vi "Dual XDCR Scan.vi"(0 "Digitizer Settings In":T27={"Digitizer delay (us) "=0.0, "rf points per line"=0, "lines per plane"=0, "Samp Rate (Hz)"=0.0, "Additional dig delay (us)"=0.0, "Voltage Scale"=0.0, "Pre-Looks"=0, "Offset delay (us)"=0.0, "bits A/D"=0, "Avg Num"=0, "DigTimeOut"=0.0, "Rel Dig Delay"=0.0, "Dig Ch"=0, "LeCroyCluster"={"LeCroy Channels"=[], "LC read pt offset"=0.0, "Sweep Avg"=FALSE}, "Main Digitizer"=enum."Acqiris Digitizer", "Dig Config"=enum."Single channel", "Digitizer ID Cluster"={"Acqiris/Alazar/SP ID"=[], "NI Instr Handles"=[], "LeCroy VISA"="", "GaGe Handle"={"Handle"=0, "Sample size"=0, "Resolution"=0, "Offset"=0, "Channels"=0, "Boards"=0}, "ATS Ref"="ATS9350", "Acqiris Address"=["PCI::INSTR0"], "ADQRef"=refnum, "adq_cu_ptr"=refnum}, "Trigger Settings"={"Trig Source"=0, "Trig Coupling"=0, "Trig Slope"=0, "Level (mV)"=0.0}, "Bulk Acq"=FALSE, "Bulk Start Indexes"=[], "Data Ref RF"=refnum, "NI ID/Channel"=[], "Total Dig CH"=1, "Xtra Ann Trig delay (us)"=10.0, "Fix Z Delay?"=FALSE, "One Way Transmission?"=FALSE, "Data Ref Log"=refnum} {"Trigger Settings"."Trig Slope" items=["Positive", "Negative"]; "Trigger Settings"."Level (mV)" format="%.2f"; "Trigger Settings"."Trig Coupling" items=["DC 1 MOhm", "AC 1 MOhm", "DC 50 Ohm", "AC 50 Ohm"]; "Trigger Settings"."Trig Source" items=["Chan 1", "External"]; "Rel Dig Delay" format="%.2f"; "DigTimeOut" format="%.2f"; "Avg Num" min=1; "Offset delay (us)" format="%.2f"; "Additional dig delay (us)" format="%.2f"; "Digitizer delay (us)" format="%.2f"}, 1 "Dual XDCR Mode":T36(ring)=enum."Exit", 3 "Motion Settings In":T31={"No Motion?"=FALSE, "Motion System"=enum."MM3000", "Motion Bd ID"=0, "Motion Profile"="SMAC1", "# Axis"=0, "Reverse Z axis?"=FALSE, "SMAC Axis"=0, "scan pair"=enum."y-(x) scan", "RT fps"=0.0, "Steps per mm"=[], "Motor Parameters"={"velocity ct/s"=[], "accel ct/s^2"=[]}, "One Way Scan"=FALSE, "Reverse One Way Scan"=FALSE, "Global Position (mm)"=[], "Plane"=0, "Distance between\nscan lines (um)"=0.0, "Distance between\nscan planes (um)"=0.0, "number of scan planes"=0, "Total steps in line"=0, "Xtra plane\ndistance  (um)"=0, "Xtra planes "=0, "Add Axis"=FALSE, "overshoot cts"=0, "BKPT Shift"=0, "Scan Start Time (ms)"=0, "ESP VISA"="", "3rd Axis"=1, "GL Ref Out"=refnum, "Galil Address"=""} {"3rd Axis" items=["x", "y", "z", "w"]; "Xtra planes" min=1; "Xtra plane\ndistance  (um)" min=0; "Distance between\nscan planes (um)" format="%.2f"; "Distance between\nscan lines (um)" format="%.2f"; "SMAC Axis" items=["None"=0, "Axis 1"=1, "Axis 2"=2, "Axis 3"=3, "Axis 4"=4, "Axis 5"=5, "Axis 6"=6, "Axis 7"=7, "Axis 8"=8, "Vector Space 1"=17, "Vector Space 2"=18, "Vector Space 3"=19, "Vector Space 4"=20]; "Motion Bd ID" min=1 max=32 step=1}, 5 "Switch Unit":T35=enum."Riverside USB", 6 "Ann Array Params":T23={"Synth Foc?"=FALSE, "Focal Zones"=41, "Switch T/R"=0, "Trans Geometry (mm)"={"Transducer"=0, "Geo Focus"=12.0, "a (radius)"=3.0, "# of rings"=5, "kerf space "=0.1, "Center Freq"=12.0}, "Sub Ap Excite?"=FALSE, "Full Array Scan?"=FALSE, "Xmt/Rcv"={"XMIT"=[TRUE, TRUE, TRUE, TRUE, TRUE], "RCV"=[TRUE, TRUE, TRUE, TRUE, TRUE]}, "PulseSpacing (us)"=0.0, "Xmit Ring"=0, "XMIT CHS"=0, "RCV CHS"=0, "GPU?"=FALSE, "Save TIFF?"=FALSE, "downfactor"=1, "RCV 1CH"=0} {"RCV 1CH" items=["All", "1", "2", "3", "4", "5"]; "Trans Geometry (mm)"."Transducer" items=["6D 12R 40 MHz"=0, "10D 31R 20 MHz"=1, "10D 23R 20 MHz"=2, "6D 23R 40 MHz"=3, "4.5D 10.7R 40 MHz"=4, "9D 23.5R 20 MHz"=5, "9D 25.8R 20MHz"=6, "Enter"=99]; "Switch T/R" min=1 max=5 step=1}, 7 "Case Name":string, 8 "Scan Parameters  Cluster":T1, 9 "Dual XDCR Settings":T2 {"XDCR Settings"."UT340 Controls"."Low Pass Filter (MHz)" min=-6 max=60 step=1; "XDCR Settings"."UT340 Controls"."High Pass Filter (MHz)" min=1 max=20 step=1; "XDCR Settings"."UT340 Controls"."Rep Rate (Hz)" min=20 step=1; "XDCR Settings"."UT340 Controls"."Pulse Width (ns)" min=100.0 max=250.0 step=2.0; "XDCR Settings"."UT340 Controls"."Voltage" min=100 max=250 step=2; "XDCR Settings"."UT340 Controls"."PC Gain (dB)" min=2 max=72; "XDCR Settings"."UT340 Controls"."PE Gain (dB)" min=-6 max=60 step=1; "XDCR Settings"."JSR Complete"."JSR Trigger Settings"."PRF (Hz)" items=["100 Hz"=0.1, "200 Hz"=0.2, "400 Hz"=0.4, "600 Hz"=0.6, "800 Hz"=0.8, "1000 Hz"=1.0, "1250 Hz"=1.25, "1500 Hz"=1.5, "1750 Hz"=1.75, "2000 Hz"=2.0, "2500 Hz"=2.5, "3000 Hz"=3.0, "3500 Hz"=3.5, "4000 Hz"=4.0, "4500 Hz"=4.5, "5000 Hz"=5.0]; "XDCR Settings"."JSR Complete"."JSR Trigger Settings"."Trigger Source" items=["Internal", "External"]; "XDCR Settings"."JSR Complete"."JSR Trigger Settings"."External Trigger Limit" items=["No Limit", "5 kHz"]; "XDCR Settings"."JSR Complete"."JSR Receive Settings"."Gain (dB)" min=-13 max=66 step=1; "XDCR Settings"."JSR Complete"."JSR Receive Settings"."Low Pass Filter" items=["5 MHz"=5, "10 MHz"=10, "15 MHz"=15, "22.5 MHz"=22, "35 MHz"=35, "50 MHz"=50]; "XDCR Settings"."JSR Complete"."JSR Receive Settings"."High Pass Filter" items=["DC"=0, "1 MHz"=1000, "2.5 MHz"=2500, "5 MHz"=5000, "7.5 MHz"=7500, "12.5 MHz"=12500]; "XDCR Settings"."JSR Complete"."JSR Receive Settings"."Receiver Mode" items=["Echo", "Through"]; "XDCR Settings"."JSR Complete"."JSR Pulse Settings"."Pulser Voltage (V)" items=["100"=100, "125"=125, "150"=150, "175"=175, "200"=200, "225"=225, "250"=250, "275"=275, "300"=300, "325"=325, "350"=350, "375"=375, "400"=400, "425"=425, "450"=450, "475"=475]; "XDCR Settings"."JSR Complete"."JSR Pulse Settings"."Pulser Impedance" items=["High z", "Low z"]; "XDCR Settings"."JSR Complete"."JSR Pulse Settings"."Pulse Energy Level" items=["0 (Minimum)", "1", "2", "3 (Maximum)"]; "XDCR Settings"."JSR Complete"."JSR Pulse Settings"."Damping" items=["331 Ohms"=331, "198 Ohms"=198, "142 Ohms"=142, "110 Ohms"=110, "92 Ohms"=92, "77 Ohms"=77, "67 Ohms"=67, "59 Ohms"=59, "52 Ohms"=52, "47 Ohms"=47, "43 Ohms"=43, "39 Ohms"=39, "37 Ohms"=37, "34 Ohms"=34, "32 Ohms"=32, "30 Ohms"=30]; "XDCR Settings"."Panametrics Settings"."FINE ATTENUATION" items=["00.0", "00.5", "01.0", "01.5", "02.0", "02.5", "03.0", "03.5", "04.0", "04.5", "05.0", "05.5", "06.0", "06.5", "07.0", "07.5", "08.0", "08.5", "09.0", "09.5", "10.0", "10.5", "11.0", "11.5", "12.0", "12.5", "13.0", "13.5", "14.0", "14.5", "15.0", "15.5"]; "XDCR Settings"."Panametrics Settings"."COARSE ATTENUATION" items=["00.0", "10.0", "20.0", "30.0", "40.0", "50.0"]; "XDCR Settings"."Panametrics Settings"."GAIN (db)" items=["26.0", "40.0", "54.0"]; "XDCR Settings"."Panametrics Settings"."PRF (KHz)" items=["XREMT", "EXBNC", "0.200", "0.500", "1.000", "2.000", "5.000", "10.00", "20.00"]; "XDCR Settings"."Panametrics Settings"."MODE" items=["P/ E", "THRU", "RPP", "EXT_PLSR"]; "XDCR Settings"."Panametrics Settings"."LP FILT (MHz)" items=["20", "50", "100", "200"]; "XDCR Settings"."Panametrics Settings"."HP FILT (KHz)" items=["1", "1000", "3000", "10000"]; "XDCR Settings"."Panametrics Settings"."DAMPING (Ohm)" items=["7", "10", "16", "20", "26", "30", "40", "50"]; "XDCR Settings"."Panametrics Settings"."ENERGY (uJ)" items=["1", "2", "4", "8", "16", "32"]; "XDCR Settings"."Daxsonics Settings"."Freq (MHz)" items=["4"=4, "5"=5, "6"=6, "8"=8, "10"=10, "12"=12, "14"=14, "15"=15, "16"=16, "17"=17, "18"=18, "20"=20, "25"=25, "30"=30, "35"=35, "40"=40, "45"=45, "50"=50]; "XDCR Settings"."Daxsonics Settings"."Voltage (V)" items=["0"=0, "5"=5, "10"=10, "15"=15, "20"=20, "25"=25, "30"=30, "35"=35, "40"=40, "45"=45, "50"=50, "55"=55, "60"=60, "65"=65, "70"=70, "75"=75, "80"=80, "85"=85, "90"=90, "95"=95, "100"=100, "110"=110, "120"=120, "130"=130, "140"=140, "150"=150, "160"=160, "170"=170, "180"=180, "190"=190]; "XDCR Settings"."Daxsonics Settings"."Gain (dB)" items=["22"=22, "25"=25, "28"=28, "31"=31, "34"=34, "37"=37, "40"=40, "43"=43, "46"=46, "49"=49, "52"=52, "55"=55, "58"=58, "61"=61, "64"=64, "67"=67]; "XDCR Settings"."Digitizer Settings"."Additional dig delay (ms)" format="%.2f"; "XDCR Settings"."Digitizer Settings"."Time scale per Div" items=["100 ns"=0.1, "200 ns"=0.2, "500 ns"=0.5, "1 micros"=1.0, "2 micros"=2.0, "5 micros"=5.0, "10 micros"=10.0, "20 micros"=20.0, "50 micros"=50.0, "100 micros"=100.0, "200 micros"=200.0, "500 micros"=500.0, "1 ms"=1000.0, "2 ms"=2000.0, "5 ms"=5000.0, "10 ms"=10000.0, "20 ms"=20000.0, "50 ms"=50000.0, "100 ms"=100000.0, "200 ms"=200000.0]; "XDCR Settings"."Digitizer Settings"."RF data Sampling"."rf points per line" min=1; "XDCR Settings"."Digitizer Settings"."RF data Sampling"."Ref Delay (ms)" format="%.2f"}) -> (12 "Ann Array Params":T23={"Synth Foc?"=FALSE, "Focal Zones"=41, "Switch T/R"=0, "Trans Geometry (mm)"={"Transducer"=0, "Geo Focus"=12.0, "a (radius)"=3.0, "# of rings"=5, "kerf space "=0.1, "Center Freq"=12.0}, "Sub Ap Excite?"=FALSE, "Full Array Scan?"=FALSE, "Xmt/Rcv"={"XMIT"=[TRUE, TRUE, TRUE, TRUE, TRUE], "RCV"=[TRUE, TRUE, TRUE, TRUE, TRUE]}, "PulseSpacing (us)"=0.0, "Xmit Ring"=0, "XMIT CHS"=0, "RCV CHS"=0, "GPU?"=FALSE, "Save TIFF?"=FALSE, "downfactor"=1, "RCV 1CH"=0} {"RCV 1CH" items=["All", "1", "2", "3", "4", "5"]; "Trans Geometry (mm)"."Transducer" items=["6D 12R 40 MHz"=0, "10D 31R 20 MHz"=1, "10D 23R 20 MHz"=2, "6D 23R 40 MHz"=3, "4.5D 10.7R 40 MHz"=4, "9D 23.5R 20 MHz"=5, "9D 25.8R 20MHz"=6, "Enter"=99]; "Switch T/R" min=1 max=5 step=1}, 13 "Case Names":string[](array[string]), 14 "Digitizer Settings":T27={"Digitizer delay (us) "=0.0, "rf points per line"=2048, "lines per plane"=128, "Samp Rate (Hz)"=100000000.0, "Additional dig delay (us)"=0.0, "Voltage Scale"=0.4, "Pre-Looks"=0, "Offset delay (us)"=0.0, "bits A/D"=8, "Avg Num"=1, "DigTimeOut"=5.0, "Rel Dig Delay"=0.0, "Dig Ch"=0, "LeCroyCluster"={"LeCroy Channels"=[TRUE, FALSE, FALSE, FALSE], "LC read pt offset"=0.0, "Sweep Avg"=FALSE}, "Main Digitizer"=enum."NI Digitizer", "Dig Config"=enum."Single channel", "Digitizer ID Cluster"={"Acqiris/Alazar/SP ID"=[], "NI Instr Handles"=[], "LeCroy VISA"="", "GaGe Handle"={"Handle"=0, "Sample size"=0, "Resolution"=0, "Offset"=0, "Channels"=0, "Boards"=0}, "ATS Ref"="ATS9350", "Acqiris Address"=["PCI::INSTR0"], "ADQRef"=refnum, "adq_cu_ptr"=refnum}, "Trigger Settings"={"Trig Source"=1, "Trig Coupling"=0, "Trig Slope"=0, "Level (mV)"=1500.0}, "Bulk Acq"=FALSE, "Bulk Start Indexes"=[], "Data Ref RF"=refnum, "NI ID/Channel"=[], "Total Dig CH"=1, "Xtra Ann Trig delay (us)"=10.0, "Fix Z Delay?"=FALSE, "One Way Transmission?"=FALSE, "Data Ref Log"=refnum} {"Trigger Settings"."Trig Slope" items=["Positive", "Negative"]; "Trigger Settings"."Level (mV)" format="%.2f"; "Trigger Settings"."Trig Coupling" items=["DC 1 MOhm", "AC 1 MOhm", "DC 50 Ohm", "AC 50 Ohm"]; "Trigger Settings"."Trig Source" items=["Chan 1", "External"]; "Rel Dig Delay" format="%.2f"; "DigTimeOut" format="%.2f"; "Avg Num" min=1; "Offset delay (us)" format="%.2f"; "Additional dig delay (us)" format="%.2f"; "Digitizer delay (us)" format="%.2f"}, 15 "Error Message":string, 17 "Motion Settings":T31={"No Motion?"=FALSE, "Motion System"=enum."NI 735x", "Motion Bd ID"=1, "Motion Profile"="SMAC1", "# Axis"=1, "Reverse Z axis?"=TRUE, "SMAC Axis"=0, "scan pair"=enum."y-(x) scan", "RT fps"=6.0, "Steps per mm"=[1000, 1000, 1000, 1000], "Motor Parameters"={"velocity ct/s"=[10000.0, 10000.0, 10000.0, 50000.0], "accel ct/s^2"=[50000.0, 50000.0, 50000.0, 200000.0]}, "One Way Scan"=FALSE, "Reverse One Way Scan"=FALSE, "Global Position (mm)"=[], "Plane"=0, "Distance between\nscan lines (um)"=0.0, "Distance between\nscan planes (um)"=0.0, "number of scan planes"=1, "Total steps in line"=0, "Xtra plane\ndistance  (um)"=100, "Xtra planes "=1, "Add Axis"=FALSE, "overshoot cts"=200, "BKPT Shift"=0, "Scan Start Time (ms)"=0, "ESP VISA"="GPIB::1::INSTR", "3rd Axis"=1, "GL Ref Out"=refnum, "Galil Address"=""} {"3rd Axis" items=["x", "y", "z", "w"]; "Xtra planes" min=1; "Xtra plane\ndistance  (um)" min=0; "Distance between\nscan planes (um)" format="%.2f"; "Distance between\nscan lines (um)" format="%.2f"; "SMAC Axis" items=["None"=0, "Axis 1"=1, "Axis 2"=2, "Axis 3"=3, "Axis 4"=4, "Axis 5"=5, "Axis 6"=6, "Axis 7"=7, "Axis 8"=8, "Vector Space 1"=17, "Vector Space 2"=18, "Vector Space 3"=19, "Vector Space 4"=20]; "Motion Bd ID" min=1 max=32 step=1}, 18 "Scan Params Array":T26[](array[typedef]), 19 "Num Scans":i32)   [LabVIEW 2022 SP3]
uses:
  Motion Controllers/NI_controller/-NI_MotionRoutines/MotionParameters.ctl
  Motion Controllers/NI_controller/-NI_MotionRoutines/MotionSys.ctl
  Motion Controllers/-MotionRoutines/ScanAxis.ctl
  Motion Controllers/-MotionRoutines/3rdAxis.ctl
  Digitizers/-DigitizerRoutines/DigitizerSettings.ctl
  Digitizers/-DigitizerRoutines/Digitizer.ctl
  Digitizers/-DigitizerRoutines/DigConfig.ctl
  Digitizers/-DigitizerRoutines/DigitizerID.ctl
  C:/Windows/System32/ADQAPI_dotNet_helper.dll
  Switch Modules/SwitchOption.ctl
  -ScanSystem/Controls/ScanParams.ctl
  Annular Array/-AnnularRoutines/AnnularArray.ctl
  Annular Array/-AnnularRoutines/TransGeometry.ctl
  Annular Array/-AnnularRoutines/ArrayGeometry.ctl
  -ScanSystem/Controls/location.ctl
  Dual XDCR Complete Settings.ctl
  XDCRSettings.ctl
  Pulsers/Daxsonics/-DaxSubroutines/Dax_Control_Cluster.ctl
  Pulsers/Panametrics/Pana5900.ctl
  Pulsers/JSR/Controls/JSR Complete.ctl
  Pulsers/JSR/Controls/JSR Pulse.ctl
  Pulsers/JSR/Controls/Damping.ctl
  Pulsers/JSR/Controls/Energy.ctl
  Pulsers/JSR/Controls/Z.ctl
  Pulsers/JSR/Controls/Volt.ctl
  Pulsers/JSR/Controls/JSR Recieve.ctl
  Pulsers/JSR/Controls/Mode.ctl
  Pulsers/JSR/Controls/HPF.ctl
  Pulsers/JSR/Controls/LPF.ctl
  Pulsers/JSR/Controls/Gain.ctl
  Pulsers/JSR/Controls/JSR Trigger.ctl
  Pulsers/JSR/Controls/Trig Limit.ctl
  Pulsers/JSR/Controls/Trig Source.ctl
  Pulsers/JSR/Controls/PRF.ctl
  Pulsers/UTEX/Controls/UTEX Controls.ctl
  -ScanSystem/Controls/ScanType2.ctl
  Motion Controllers/-MotionRoutines/MotionGlobals.vi
  Pulsers/PulserGlobals.vi
  <instrlib>/niSwitch/niSwitch.llb/niSwitch Connect Channels (Single).vi
panel:
  out "Location":T22=enum."WCM Main"
  out "One Way Scan":bool
  # "1-D and 2-D B scan settings"
  # "1-D and 2-D B scan settings"
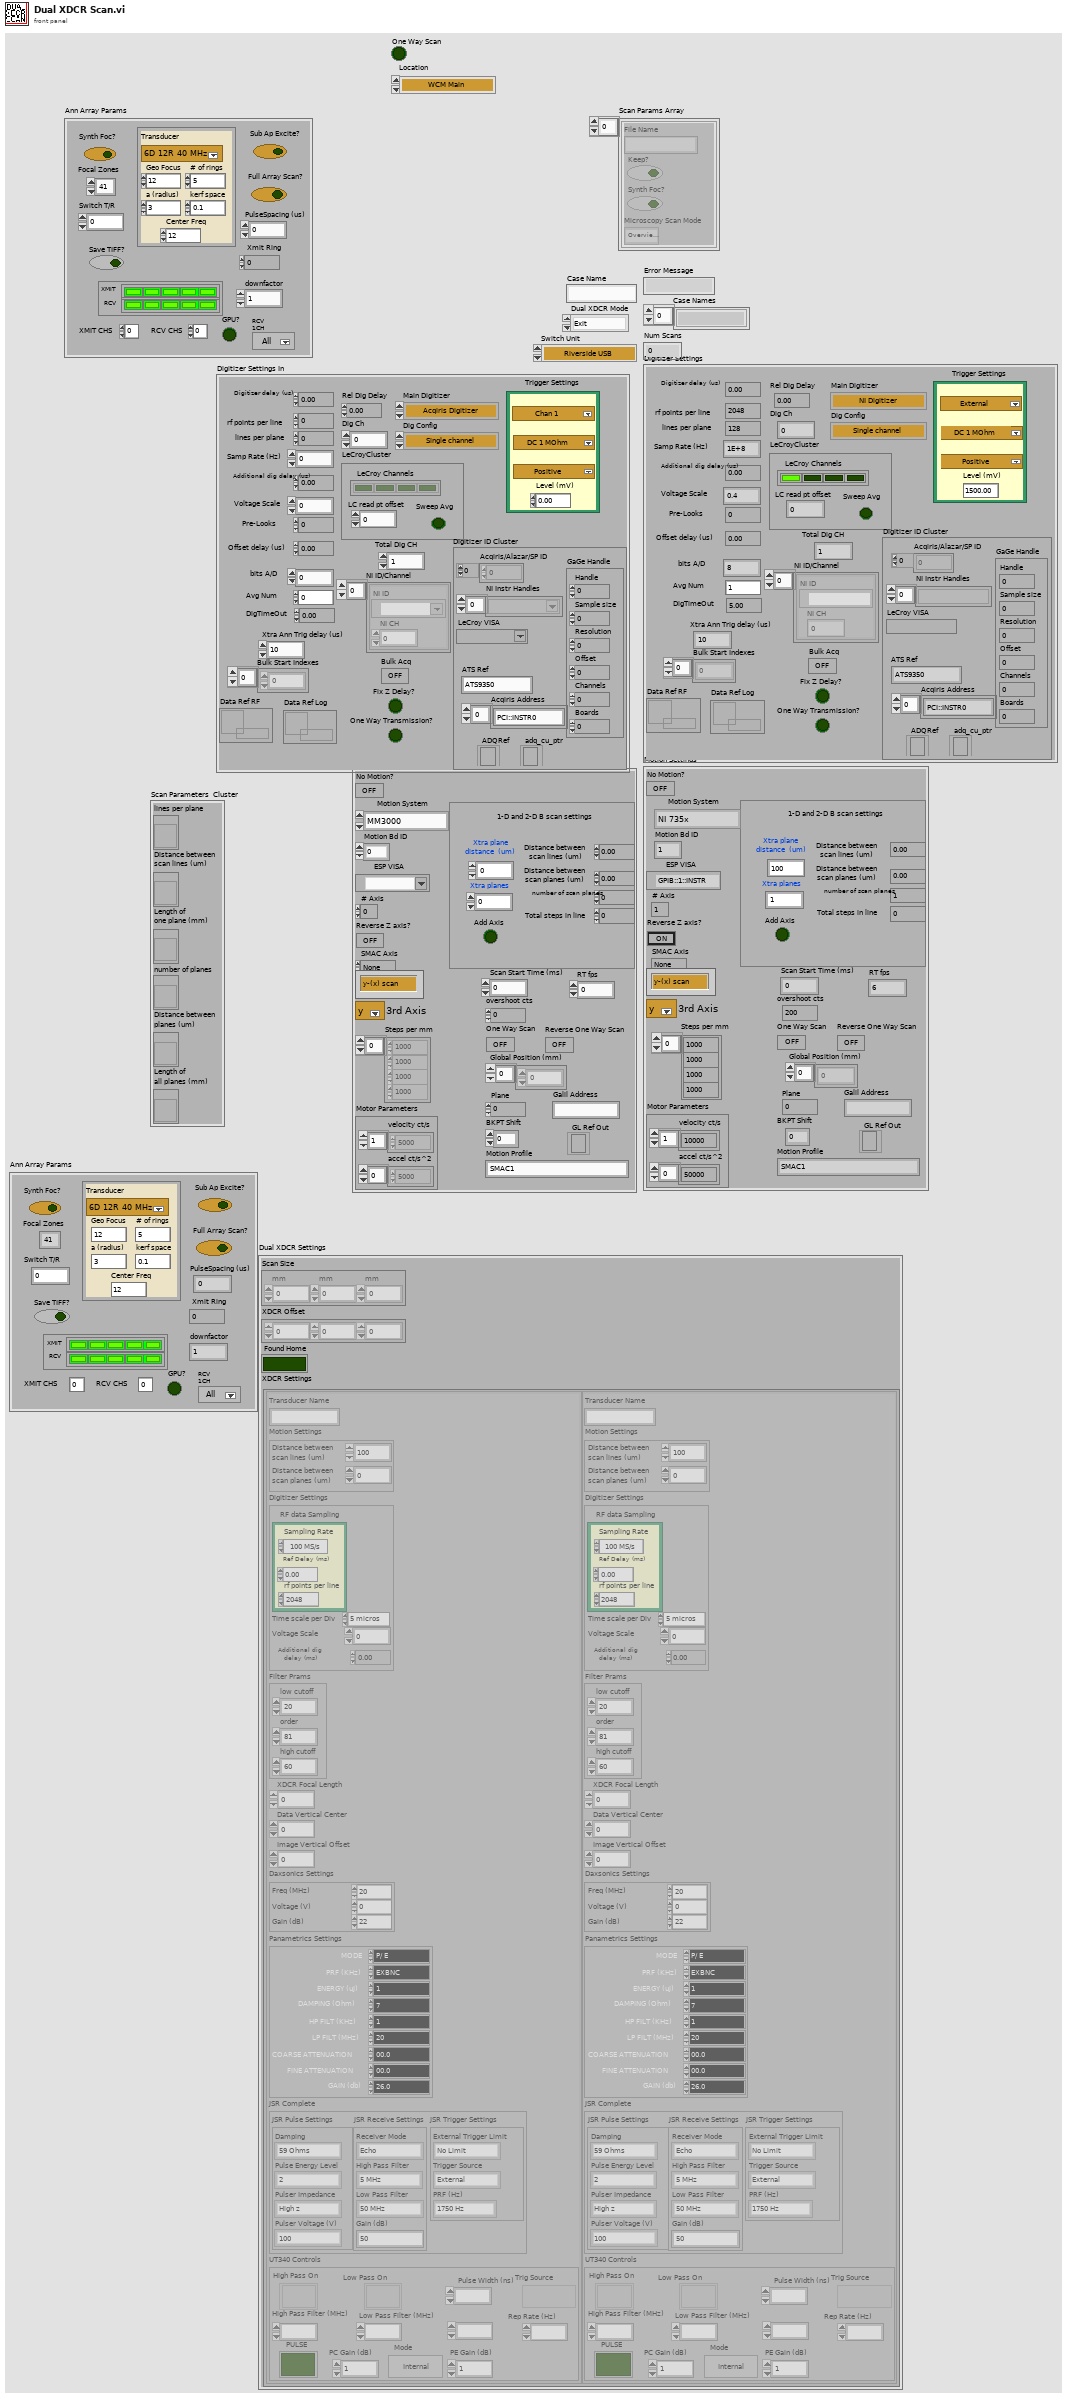
[diagram p1: front panel]
types:
  T1 = cluster{"lines per plane":refnum<vi>, "Distance between\nscan lines (um)":refnum<vi>, "Length of\none plane (mm)":refnum<vi>, "number of planes":refnum<vi>, "Distance between\nplanes (um)":refnum<vi>, "Length of\nall planes (mm)":refnum<vi>}
  T2 = typedef "Dual XDCR Complete Settings.ctl" = cluster{"Scan Size":dbl[], "XDCR Offset":dbl[], "Found Home":bool, "XDCR Settings":T3[]}
  T3 = typedef "XDCRSettings.ctl" = cluster{"Transducer Name":string, "Motion Settings":cluster{"Distance between\nscan lines (um)":sgl, "Distance between\nscan planes (um)":sgl}, "Digitizer Settings":cluster{"RF data Sampling":cluster{"Sampling Rate":dbl, "Ref Delay (ms)":dbl, "rf points per line":i32}, "Time scale per Div":dbl, "Voltage Scale":dbl, "Additional dig delay (ms)":dbl}, "Filter Prams":cluster{"low cutoff":i32, "order":i32, "high cutoff":i32}, "XDCR Focal Length":dbl, "Data Vertical Center":dbl, "Image Vertical Offset":dbl, "Daxsonics Settings":T4, "Panametrics Settings":T5, "JSR Complete":T6, "UT340 Controls":T21}
  T4 = typedef "Dax_Control_Cluster.ctl" = cluster{"Freq (MHz) ":u16, "Voltage (V)":u16, "Gain (dB)":u16}
  T5 = typedef "Pana5900.ctl" = cluster{"ENERGY (uJ)":u16, "DAMPING (Ohm)":u16, "HP FILT (KHz) ":u16, "LP FILT (MHz)":u16, "MODE":u16, "PRF (KHz)":u16, "GAIN (db)":u16, "COARSE ATTENUATION":u16, "FINE ATTENUATION":u16}
  T6 = typedef "JSR Complete.ctl" = cluster{"JSR Pulse Settings":T7, "JSR Receive Settings":T12, "JSR Trigger Settings":T17}
  T7 = typedef "JSR Pulse.ctl" = cluster{"Damping":T8, "Pulse Energy Level":T9, "Pulser Impedance":T10, "Pulser Voltage (V)":T11}
  T8 = typedef "Damping.ctl" = i16
  T9 = typedef "Energy.ctl" = u16
  T10 = typedef "Z.ctl" = u16
  T11 = typedef "Volt.ctl" = i16
  T12 = typedef "JSR Recieve.ctl" = cluster{"Receiver Mode":T13, "High Pass Filter":T14, "Low Pass Filter":T15, "Gain (dB)":T16}
  T13 = typedef "Mode.ctl" = i8
  T14 = typedef "HPF.ctl" = u16
  T15 = typedef "LPF.ctl" = u16
  T16 = typedef "Gain.ctl" = i8
  T17 = typedef "JSR Trigger.ctl" = cluster{"External Trigger Limit":T18, "Trigger Source":T19, "PRF (Hz)":T20}
  T18 = typedef "Trig Limit.ctl" = i8
  T19 = typedef "Trig Source.ctl" = i8
  T20 = typedef "PRF.ctl" = dbl
  T21 = typedef "UTEX Controls.ctl" = cluster{"High Pass On":bool, "High Pass Filter (MHz)":i16, "Low Pass On":bool, "Low Pass Filter (MHz)":i16, "PE Gain (dB)":i16, "Voltage":i16, "Pulse Width (ns)":dbl, "Mode":bool, "PC Gain (dB)":i16, "Trig Source":bool, "Rep Rate (Hz)":i16, "PULSE":bool}
  T22 = typedef "location.ctl" = enum16{"Automatic", "WCM Main", "Hawaii", "Columbia MM3000", "Columbia  NI System", "NYU", "RRI 2", "UHI Allen", "CUMC RT", "Chiba", "Stony Brook", "WCM Microscopy", "WCM Aeoretch", "WCM Optics Lab", "WCM Main 2Axis", "WCM Rotation", "WCM SAM SMAC", "SERI GP"}
  T23 = typedef "AnnularArray.ctl" = cluster{"Synth Foc?":bool, "Focal Zones":i16, "Switch T/R":i16, "Trans Geometry (mm)":T24, "Sub Ap Excite?":bool, "Full Array Scan?":bool, "Xmt/Rcv":cluster{"XMIT":bool[], "RCV":bool[]}, "PulseSpacing (us)":sgl, "Xmit Ring":i32, "XMIT CHS":u8, "RCV CHS":u8, "GPU?":bool, "Save TIFF?":bool, "downfactor":i32, "RCV 1CH":u16}
  T24 = typedef "TransGeometry.ctl" = cluster{"Transducer":T25, "Geo Focus":dbl, "a (radius)":dbl, "# of rings":i32, "kerf space ":dbl, "Center Freq":dbl}
  T25 = typedef "ArrayGeometry.ctl" = u16
  T26 = typedef "ScanParams.ctl" = cluster{"File Name":string, "Keep?":bool, "Synth Foc?":bool, "Microscopy Scan Mode":enum32{"Level X", "Level Y", "Overview Scan", "Detailed Scan", "V-Z Scan"}}
  T27 = typedef "DigitizerSettings.ctl" = cluster{"Digitizer delay (us) ":dbl, "rf points per line":i32, "lines per plane":i32, "Samp Rate (Hz)":dbl, "Additional dig delay (us)":dbl, "Voltage Scale":dbl, "Pre-Looks":i32, "Offset delay (us)":dbl, "bits A/D":i8, "Avg Num":i32, "DigTimeOut":sgl, "Rel Dig Delay":sgl, "Dig Ch":i32, "LeCroyCluster":cluster{"LeCroy Channels":bool[], "LC read pt offset":dbl, "Sweep Avg":bool}, "Main Digitizer":T28, "Dig Config":T29, "Digitizer ID Cluster":T30, "Trigger Settings":cluster{"Trig Source":u16, "Trig Coupling":u16, "Trig Slope":u16, "Level (mV)":dbl}, "Bulk Acq":bool, "Bulk Start Indexes":i32[], "Data Ref RF":refnum<data-value>, "NI ID/Channel":cluster{"NI ID":refnum<k15>, "NI CH":i32}[], "Total Dig CH":i32, "Xtra Ann Trig delay (us)":dbl, "Fix Z Delay?":bool, "One Way Transmission?":bool, "Data Ref Log":refnum<data-value>}
  T28 = typedef "Digitizer.ctl" = enum16{"Acqiris Digitizer", "NI Digitizer", "LeCroy", "GaGe", "AlazarTech", "No Digitizer", "Teledyne"}
  T29 = typedef "DigConfig.ctl" = enum16{"Single channel", "2 Chans w/ 2 Acqiris", "2 Chans w/ 1 Acqiris", "5-CH Pulser New", "5-CH pulser w/ ann array", "5-pass style ann array", "Empty"}
  T30 = typedef "DigitizerID.ctl" = cluster{"Acqiris/Alazar/SP ID":u32[], "NI Instr Handles":refnum<k15>[], "LeCroy VISA":refnum<visa-resource-name>, "GaGe Handle":cluster{"Handle":u32, "Sample size":u32, "Resolution":i32, "Offset":i32, "Channels":u32, "Boards":u32}, "ATS Ref":string, "Acqiris Address":string[], "ADQRef":refnum<k24>, "adq_cu_ptr":refnum<k24>}
  T31 = typedef "MotionParameters.ctl" = cluster{"No Motion?":bool, "Motion System":T32, "Motion Bd ID":u8, "Motion Profile":string, "# Axis":i8, "Reverse Z axis?":bool, "SMAC Axis":u16, "scan pair":T33, "RT fps":sgl, "Steps per mm":i32[], "Motor Parameters":cluster{"velocity ct/s":dbl[], "accel ct/s^2":dbl[]}, "One Way Scan":bool, "Reverse One Way Scan":bool, "Global Position (mm)":dbl[], "Plane":i32, "Distance between\nscan lines (um)":sgl, "Distance between\nscan planes (um)":sgl, "number of scan planes":i32, "Total steps in line":i32, "Xtra plane\ndistance  (um)":i32, "Xtra planes ":i32, "Add Axis":bool, "overshoot cts":i32, "BKPT Shift":i32, "Scan Start Time (ms)":u32, "ESP VISA":refnum<visa-resource-name>, "3rd Axis":T34, "GL Ref Out":refnum<k7>, "Galil Address":string}
  T32 = typedef "MotionSys.ctl" = enum16{"MM3000", "NI 735x", "Newport ESP", "No Motion Card", "Galil"}
  T33 = typedef "ScanAxis.ctl" = enum16{"y-(x) scan", "x-(y) scan", "z-(x) scan", "z-(y) scan", "y-(z) scan", "x-(z) scan", "w-(x) scan", "w-(y) scan", "w-(z) scan", "x-(w) scan", "y-(w) scan", "z-(w) scan"}
  T34 = typedef "3rdAxis.ctl" = u16
  T35 = typedef "SwitchOption.ctl" = enum16{"Cytex", "Pickering", "NI Switch", "No Switch", "Riverside USB"}
  T36 = enum16{"Transducer 1", "Transducer 2", "Dual XDCR", "Exit"}
  T37 = typedef "pulser.ctl" = enum16{"Pan 5900", "Daxsonics", "Agilent 33xxx", "UTEX", "JSR", "WMC Mono-Cycle", "No Pulser", "NYU AVTECH", "Tabor W1281A", "Pan 5800", "Unlisted", "Tabor WX2182B"}
  T38 = enum16{"Absolute Position", "Relative Position", "Velocity", "Relative to Cap Pos", "Modulus Position", "Absolute Contouring", "Relative Contouring"}
  T39 = typedef "ScanType2.ctl" = enum16{"Therapy With Scan", "M scan", "M Scan With Therapy Burst", "1-D B Scan", "1-D B Scan With Therapy Burst", "2-D B Scan", "2-D B Scan With Therapy Burst", "Rotational Scan", "1-D B-Scan PRF", "2-D B-Scan PRF", "Real-Time Scan", "Contrast Agents", "1-D w/ Real-Time Set Up", "Dual Transducer", "Acoustic Microscopy", "Hydrophone Scanning"}
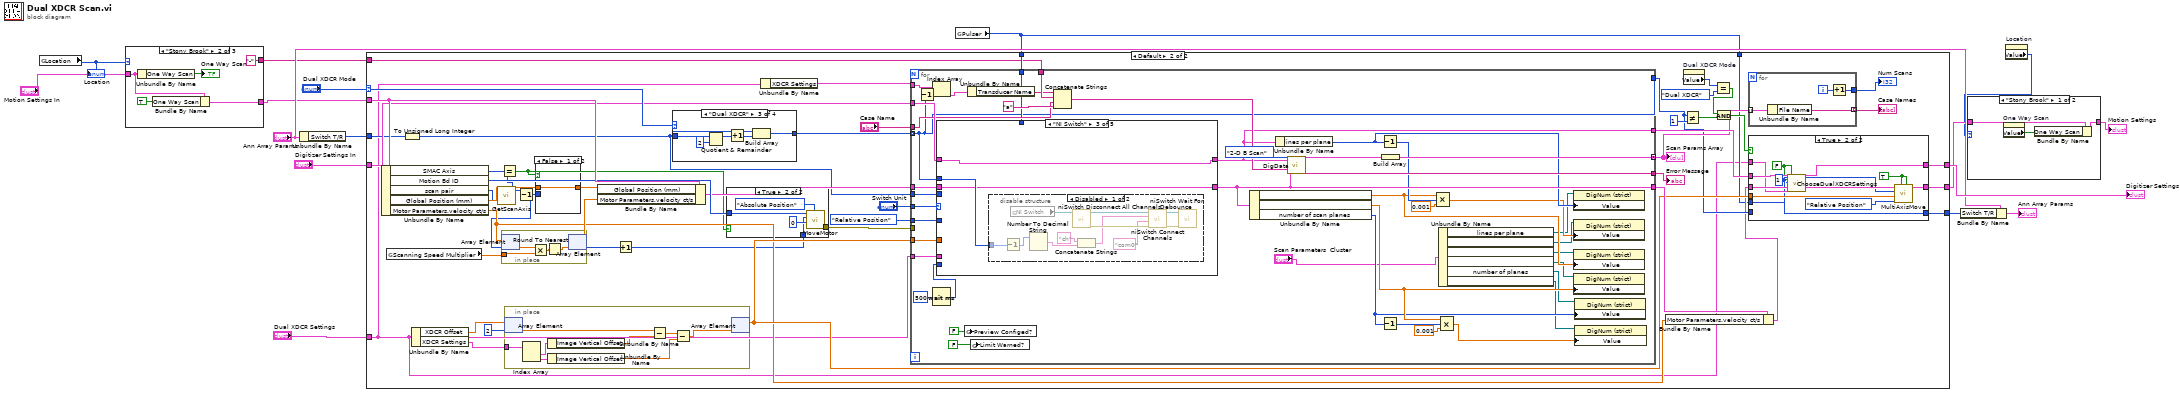
[diagram p0: block diagram]
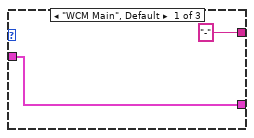
[diagram p3: hidden frame]
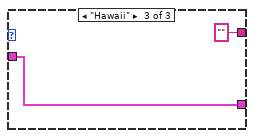
[diagram p4: hidden frame]
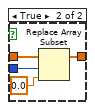
[diagram p6: hidden frame]
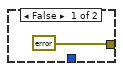
[diagram p7: hidden frame]
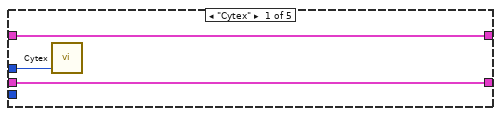
[diagram p9: hidden frame]
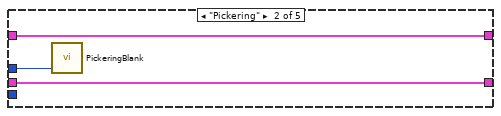
[diagram p10: hidden frame]
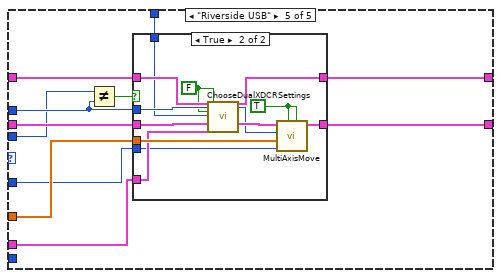
[diagram p13: hidden frame]
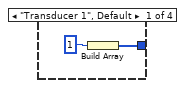
[diagram p15: hidden frame]
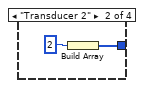
[diagram p16: hidden frame]
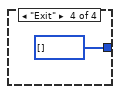
[diagram p17: hidden frame]
diagram:
  n1 = global read "MotionGlobals.vi" "Location"() -> (w6:T22)
  "Location" <- w6
  n2 = case shown="\"Stony Brook\"" w6 {
    tunnel: "Motion Settings In" -> [w18 w22 w25]
    tunnel: [w18 w20 w25] -> w5
    tunnel: ["-" ("string") "-" ("string") "" ("string")] -> w2
    frame "WCM Main", Default {
    }
    frame "Stony Brook" {
      n3 = Unbundle By Name(w22) -> ("One Way Scan"=→"One Way Scan":bool)
      n4 = Bundle By Name(cluster=w22, "One Way Scan"=TRUE) -> (w20:T31)
    }
    frame "Hawaii" {
    }
  }
  n5 = Unbundle By Name("Ann Array Params") -> ("Switch T/R"=w13:i16)
  n6 = global read "PulserGlobals.vi" "Pulser"() -> (w3:T37)
  n7 = case shown="Default" "Dual XDCR Mode" {
    selector: "Dual XDCR Mode" -> [_ w66]
    tunnel: w5 -> [w28 w73]
    tunnel: "Digitizer Settings In" -> [w27 w65]
    tunnel: [w27 w64] -> w14
    tunnel: [w28 w63] -> w7
    tunnel: "Dual XDCR Settings" -> [_ w37]
    tunnel: [w26 w50] -> w10
    tunnel: w13 -> [w26 w48]
    tunnel: w3 -> [_ w41]
    tunnel: w3 -> [_ w40]
    tunnel: w2 -> [_ w38]
    frame "Exit" {
    }
    frame Default {
      n8 = Unbundle By Name(w73) -> ("SMAC Axis"=w31:u16, "Motion Bd ID"=w71:u8, "scan pair"=w42:T33, "Global Position (mm)"=w72:dbl[], "Motor Parameters.velocity ct/s"=w44:dbl[])
      n9 = global read "MotionGlobals.vi" "Scanning Speed Multiplier"() -> (w43:dbl)
      n10 = To Unsigned Long Integer(number=w48) -> (unsigned 32bit integer=w30:u32)
      n11 = Unbundle By Name(w37) -> ("XDCR Offset"=w60:dbl[], "XDCR Settings"=w58:T3[])
      n12 = call "GetScanAxis.vi"("scan pair"=w42) -> ("Axis 1"=w32:i32)  [unwired: 1 in, 2 out]
      n13 = Equal?(x=w31, y=w32) -> (x = y?=w29:bool)
      n14 = in-place {
        in-place-border: w58 -> [w96]
        n15 = in-place-array #1(w60, 2) -> (w95:dbl)
        n16 = Index Array(array=w96) -> (element #1=w100:T3, element #2=w101:T3)  [unwired: 2 in]
        n17 = Unbundle By Name(w100) -> ("Image Vertical Offset"=w99:dbl)
        n18 = Unbundle By Name(w101) -> ("Image Vertical Offset"=w97:dbl)
        n19 = Subtract(x=w95, y=w99) -> (x-y=w98:dbl)
        n20 = Subtract(x=w98, y=w97) -> (x-y=w94:dbl)
        n21 = in-place-array #1(w94) -> (w57:dbl[])  [unwired: 1 out]
      }
      n22 = Decrement(x=w32) -> (x-1=w35:i32)
      n23 = in-place {
        in-place-border: w43 -> [w90]
        n24 = in-place-array #2(w44, w35) -> (w93:dbl)
        n25 = Multiply(x=w93, y=w90) -> (x*y=w92:dbl)
        n26 = Round To Nearest(number=w92) -> (nearest integer value=w91:dbl)
        n27 = in-place-array #2(w91) -> (w46:dbl[], w34:i32)
      }
      n28 = case shown="False" w29 {
        tunnel: w72 -> [w79 w83]
        tunnel: [w79 w81] -> w61
        tunnel: w35 -> [_ w80]
        frame False {
        }
        frame True {
          n29 = Replace Array Subset(array=w83, new element=0.0 ("new element/subarray"), index=w80) -> (w81:dbl[])
        }
      }
      n30 = Bundle By Name(cluster=w73, "Global Position (mm)"=w61, "Motor Parameters.velocity ct/s"=w46) -> (w47:T31)
      n31 = Increment(x=w34) -> (x+1=w33:i32)
      n32 = case shown="\"Dual XDCR\"" w66 {
        tunnel: w30 -> [_ _ w221 _]
        tunnel: [w214 w216 w218 u32[] []] -> w39
        frame "Transducer 1", Default {
          n33 = Build Array(1) -> (w214:i32[])
        }
        frame "Transducer 2" {
          n34 = Build Array(2) -> (w216:i32[])
        }
        frame "Dual XDCR" {
          n35 = Quotient & Remainder(x=w221, y=u32 2) -> (x-y*floor(x/y)=w220:u32)  [unwired: 1 out]
          n36 = Increment(x=w220) -> (x+1=w219:u32)
          n37 = Build Array(w221, w219) -> (w218:u32[])
        }
        frame "Exit" {
        }
      }
      n38 = case shown="True" w29 {
        tunnel: w71 -> [_ w89]
        tunnel: [errorcluster {"status"=FALSE, "code"=0, "source"=""} ("error out") w86] -> w70
        tunnel: w33 -> [_ w85]
        frame False {
        }
        frame True {
          n39 = call "MoveMotor.vi"("Position Mode (Absolute)"=T38."Absolute Position", "Target Position (0)"=0 ("Primary Reset Position (0)"), "Axis or Vector Space"=w85, "Motion Bd ID"=w89) -> ("error out"=w86:errorcluster)  [unwired: 5 in, 2 out]
        }
      }
      n40 = Unbundle By Name(w37) -> ("XDCR Settings"=w36:T3[])
      n41 = for {
        tunnel: w57 -> [w164]
        tunnel: w65 -> [w163]
        tunnel: w47 -> [w162]
        tunnel: "Case Name" -> [w152]
        tunnel: "Switch Unit" -> [w160]
        tunnel: w39 -> [w130] mode=indexing
        tunnel: [w159] -> w69 mode=concatenating
        tunnel: [w150] -> w75
        tunnel: [w151] -> w74
        tunnel: [w158] -> w76
        tunnel: w30 -> [w157]
        tunnel: w70 -> [_]
        tunnel: w37 -> [w154]
        tunnel: T38."Relative Position" ("Position Mode (Absolute)") -> [w153]
        tunnel: [w130] -> w49
        tunnel: w40 -> [w133]
        tunnel: w36 -> [w131]
        tunnel: w38 -> [w132]
        n42 = Decrement(x=w130) -> (x-1=w129:u32)
        n43 = Index Array(array=w131, index=w129) -> (element=w128:T3)
        n44 = Wait (ms)(milliseconds to wait=u32 500) -> (millisecond timer value=w124:u32)
        n45 = case shown="\"NI Switch\"" w160 {
          tunnel: [w167 w170 w173 w187 w197] -> w150
          tunnel: [w166 w169 w172 w186 w198] -> w151
          tunnel: w164 -> [_ _ _ _ w196]
          tunnel: w163 -> [w167 w170 w173 w187 w195]
          tunnel: w162 -> [w166 w169 w172 w186 w194]
          tunnel: w130 -> [w168 w171 w174 _ w193]
          tunnel: w157 -> [_ _ _ _ w192]
          tunnel: w154 -> [_ _ _ _ w190]
          tunnel: w153 -> [_ _ _ _ w189]
          tunnel: w133 -> [_ _ _ _ w188]
          tunnel: w124 -> [_ _ _ _ _]
          frame "Cytex" {
            n46 = call "Cytex.vi"("Xmit Ring"=w168) -> ()  [unwired: 2 in, 3 out]
          }
          frame "Pickering" {
            n47 = call "PickeringBlank.vi"("Xmit Ring"=w171) -> ()  [unwired: 5 out]
          }
          frame "NI Switch" {
            n48 = disable-structure shown="Disabled" {
              disable-tunnel: w174 -> [w175 _]
              frame Disabled {
                n49 = Decrement(x=w175) -> (x-1=w185:u32)
                n50 = global read "MotionGlobals.vi" "NI Switch"() -> (w178:refnum<k15>)
                n51 = Number To Decimal String(number=w185) -> (decimal integer string=w184:string)  [unwired: 1 in]
                n52 = call <instrlib>:"niSwitch Disconnect All Channels.vi"("instrument handle"=w178) -> ("error out"=w180:errorcluster, "instrument handle out"=w179:refnum<k15>)  [unwired: 9 in]
                n53 = Concatenate Strings("ch", w184) -> (w176:string)
                n54 = call-poly <instrlib>:"niSwitch Connect Channels.vi"("error in (no error)"=w180, "channel 2"="com0", "channel 1"=w176, "instrument handle"=w179) -> ("error out"=w181:errorcluster, "instrument handle out"=w182:refnum<k15>)  [unwired: 6 in]
                n55 = call <instrlib>:"niSwitch Wait For Debounce.vi"("error in (no error)"=w181, "instrument handle"=w182) -> ()  [unwired: 8 in, 2 out]
              }
              frame Enabled {
              }
            }
          }
          frame "No Switch", Default {
          }
          frame "Riverside USB" {
            n56 = Not Equal?(x=w192, y=w193) -> (x != y?=w191:bool)
            n57 = case shown="True" w191 {
              tunnel: [w200 w213] -> w197
              tunnel: [w199 w204] -> w198
              tunnel: w196 -> [_ w210]
              tunnel: w195 -> [w200 w209]
              tunnel: w194 -> [w199 w208]
              tunnel: w193 -> [_ w207]
              tunnel: w190 -> [_ w206]
              tunnel: w189 -> [_ w205]
              tunnel: w188 -> [_ w202]
              frame False {
              }
              frame True {
                w203 = TRUE ("Wait For Move Complete")
                w201 = FALSE ("Setup Time\nParameters (F)")
                n58 = call "ChooseDualXDCRSettings.vi"("Digitizer Settings in"=w209, "Switch T/R"=w207, "Set All UTEX?"=w201, "Pulser"=w202, "Motion Settings in"=w208, "Dual XDCR Settings"=w206, "Setup Time\nParameters (F)"=w201) -> ("Digitizer Settings"=w213:T27, "Change Polarity"=w211:i32, "Motion Settings"=w212:T31)  [unwired: 18 in]
                n59 = call "MultiAxisMove.vi"("Find Location"=w203, "Wait For Move Complete"=w203, "Position Mode (Rel)"=w205, "Distance to move (mm)"=w210, "Move Polarity"=w211, "Motion Settings"=w212) -> ("Motion Settings Out"=w204:T31)  [unwired: 3 in, 2 out]
              }
            }
          }
        }
        n60 = global write "MotionGlobals.vi" "Preview Configed?"(FALSE ("Popped Up Before?")) -> ()
        n61 = Unbundle By Name(w128) -> ("Transducer Name"=w127:string)
        n62 = global write "MotionGlobals.vi" "Limit Warned?"(FALSE ("Popped Up Before?")) -> ()
        n63 = Concatenate Strings(w127, w132, w152, "a" ("string")) -> (w156:string)
        n64 = Unbundle By Name(w151) -> ("Distance between\nscan lines (um)"=w141:sgl, "Distance between\nscan planes (um)"=w149:sgl, "number of scan planes"=w148:i32)
        n65 = Unbundle By Name(w150) -> ("lines per plane"=w142:i32)
        n66 = call "DigData.vi"("Type of scan"=ScanType2."2-D B Scan", "Digitizer Settings"=w150, "File Name In"=w156, "Motion Settings In"=w151) -> ("Scan Params"=w165:T26, "Error Message"=w158:string)  [unwired: 11 in, 11 out]
        n67 = Decrement(x=w142) -> (x-1=w143:i32)
        n68 = Decrement(x=w148) -> (x-1=w146:i32)
        n69 = Build Array(w165) -> (w159:T26[])
        n70 = Compound Arithmetic op=MULTIPLY(w141, w143, 0.001 ("value")) -> (w140:dbl)
        n71 = Unbundle By Name("Scan Parameters  Cluster") -> ("lines per plane"=w139:refnum<vi>, "Length of\none plane (mm)"=w138:refnum<vi>, "Distance between\nscan lines (um)"=w137:refnum<vi>, "Distance between\nplanes (um)"=w136:refnum<vi>, "number of planes"=w135:refnum<vi>, "Length of\nall planes (mm)"=w134:refnum<vi>)
        n72 = Compound Arithmetic op=MULTIPLY(w149, w146, 0.001 ("value")) -> (w145:dbl)
        n73 = property class="DigNum (strict)"(reference=w139, "Value"=w142) -> ()  [unwired: 1 in, 2 out]
        n74 = property class="DigNum (strict)"(reference=w138, "Value"=w140) -> ()  [unwired: 1 in, 2 out]
        n75 = property class="DigNum (strict)"(reference=w137, "Value"=w141) -> ()  [unwired: 1 in, 2 out]
        n76 = property class="DigNum (strict)"(reference=w136, "Value"=w149) -> ()  [unwired: 1 in, 2 out]
        n77 = property class="DigNum (strict)"(reference=w135, "Value"=w148) -> ()  [unwired: 1 in, 2 out]
        n78 = property class="DigNum (strict)"(reference=w134, "Value"=w145) -> ()  [unwired: 1 in, 2 out]
      }
      "Scan Params Array" <- w69
      "Error Message" <- w76
      n79 = Bundle By Name(cluster=w74, "Motor Parameters.velocity ct/s"=w44) -> (w45:T31)
      n80 = property on="Dual XDCR Mode" class="Enum (strict)"() -> ("Value"=w53:T36)  [unwired: 2 in, 2 out]
      n81 = Not Equal?(x=w49, y=u32 1) -> (x != y?=w55:bool)
      n82 = Equal?(x=w53, y=T36."Dual XDCR") -> (x = y?=w52:bool)
      n83 = And(x=w52, y=w55) -> (x .and. y?=w54:bool)
      n84 = for {
        tunnel: [w102] -> w67
        tunnel: [w104] -> w68 mode=indexing
        tunnel: w69 -> [w103] mode=indexing
        i -> [w105]
        n85 = Unbundle By Name(w103) -> ("File Name"=w104:string)
        n86 = Increment(x=w105) -> (x+1=w102:i32)
      }
      "Case Names" <- w68
      "Num Scans" <- w67
      n87 = case shown="True" w54 {
        tunnel: [w108 w121] -> w64
        tunnel: [w107 w118] -> w63
        tunnel: w75 -> [w108 w117]
        tunnel: w45 -> [w107 w116]
        tunnel: w57 -> [_ w115]
        tunnel: w37 -> [_ w114]
        tunnel: [w106 w111] -> w50
        tunnel: w49 -> [w106 _]
        tunnel: w41 -> [_ w110]
        frame False {
        }
        frame True {
          w111 = u32 1 ("Switch T/R")
          w109 = FALSE ("Setup Time\nParameters (F)")
          w112 = TRUE ("Find Location")
          n88 = call "ChooseDualXDCRSettings.vi"("Digitizer Settings in"=w117, "Switch T/R"=w111, "Set All UTEX?"=w109, "Pulser"=w110, "Motion Settings in"=w116, "Dual XDCR Settings"=w114, "Setup Time\nParameters (F)"=w109) -> ("Digitizer Settings"=w121:T27, "Change Polarity"=w119:i32, "Motion Settings"=w120:T31)  [unwired: 18 in]
          n89 = call "MultiAxisMove.vi"("Find Location"=w112, "Wait For Move Complete"=w112, "Position Mode (Rel)"=T38."Relative Position" ("Position Mode (Absolute)"), "Distance to move (mm)"=w115, "Move Polarity"=w119, "Motion Settings"=w120) -> ("Motion Settings Out"=w118:T31)  [unwired: 3 in, 2 out]
        }
      }
    }
  }
  "Digitizer Settings" <- w14
  n90 = Bundle By Name(cluster="Ann Array Params", "Switch T/R"=w10) -> (→"Ann Array Params":T23)
  n91 = property on="Location" class="Enum (strict)"() -> ("Value"=w4:T22)  [unwired: 2 in, 2 out]
  n92 = case shown="\"Stony Brook\"" w4 {
    tunnel: [w225 w227] -> w8
    tunnel: w7 -> [w226 w227]
    frame "Stony Brook" {
      n93 = property on="One Way Scan" class="Bool (strict)"() -> ("Value"=w224:bool)  [unwired: 2 in, 2 out]
      n94 = Bundle By Name(cluster=w226, "One Way Scan"=w224) -> (w225:T31)
    }
    frame "WCM Main", Default {
    }
  }
  "Motion Settings" <- w8
